vi "1 Optical Motion (with Velocity Plot).vi"() -> ()   [LabVIEW 2012]
doc: "This example shows how to use the Lucas Kanade Pyramid motion estimation VI to track features in a sequence of images in NI Vision. The VI reads the frames from an AVI file and tracks user specified features in the image from frame to frame."
uses:
  <vilib>/userdefined/High Color/IMAQdx.ctl
  <vilib>/vision/driver/NI_Vision_Acquisition_Software.lvlib
  <vilib>/vision/NI_Vision_Development_Module.lvlib
panel:
  out "Distance Array":dbl[](array[slide])=[0.2733994049757765, 0.23499957403887414, 0.19572823579546908, 0.3099445751011246, 0.800848062565794, 0.07985501092672606, 0.034294158969479405, 0.2777074897572326, 0.19929800724297095, 0.1271143119257122, 0.21415195112343915, 0.28639636417045206, 0.3114689873551136, 0.07118602059901899] caption="DistanceArray" scale=0.0..40.0
  in  "Select Points":bool caption="Click on the image and select the points to track. Press the <Ctrl> key while selecting  multiple points. Press the  \"Select Points\" button after  all points have been selected."
  in  "Options":T1={"Level"=4, "maxiteration"=20, "windowsize"=20, "threshold"=1.0}
  out "Image":T2(plugin-control)
  in  "Stop":bool
  # "My iphone is low resolution. You may need\nto experiment with these setting to make it\nwork correctly with your camera. Start by \ntweeking the Window Size"
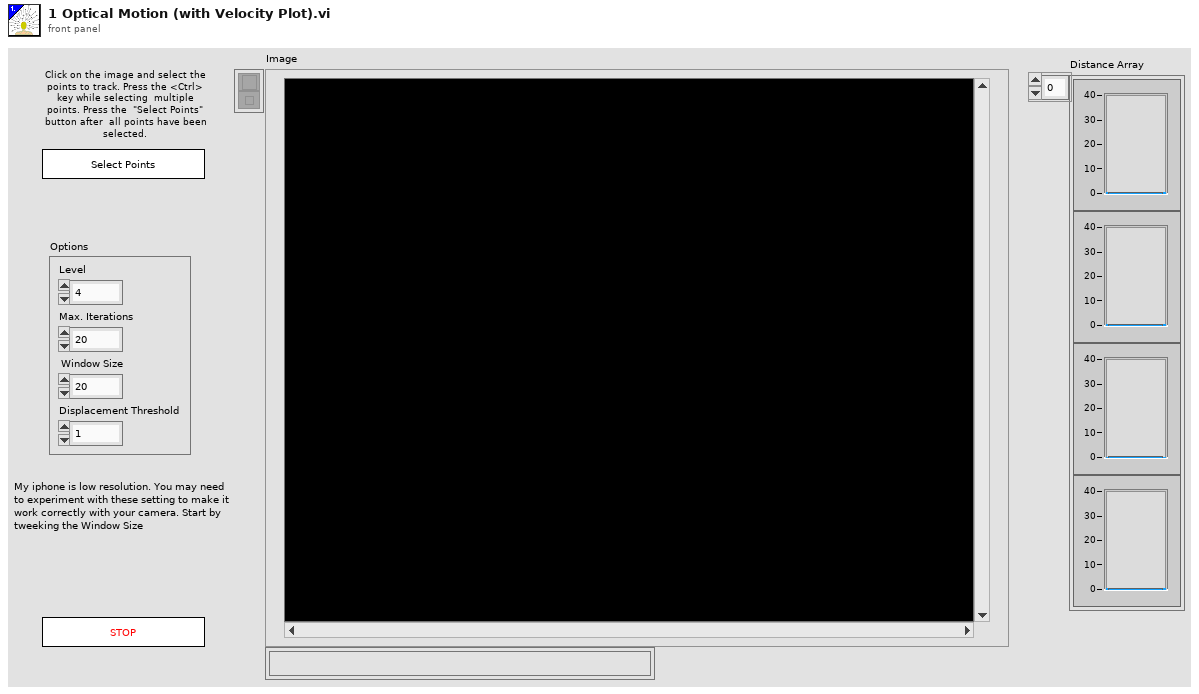
[diagram p1: front panel]
types:
  T1 = cluster{"Level":i32, "maxiteration":i32, "windowsize":i32, "threshold":dbl}
  T2 = typedef "IMAQ Image.ctl" = refnum<image>
  T3 = typedef "IMAQdx.ctl" = refnum<k21>
  T4 = cluster{"Global Rectangle":i32[], "Contours":cluster{"Contour Type":u32, "ROI Type":u32, "Points":i32[]}[]}
  T5 = typedef "ROI Descriptor" = cluster{"Global Rectangle":i32[], "Contours":cluster{"ID":enum32{"External", "Internal"}, "Type":u32, "Coordinates":i32[]}[]}
  T6 = typedef "IMAQ Point" = cluster{"X":sgl, "Y":sgl}
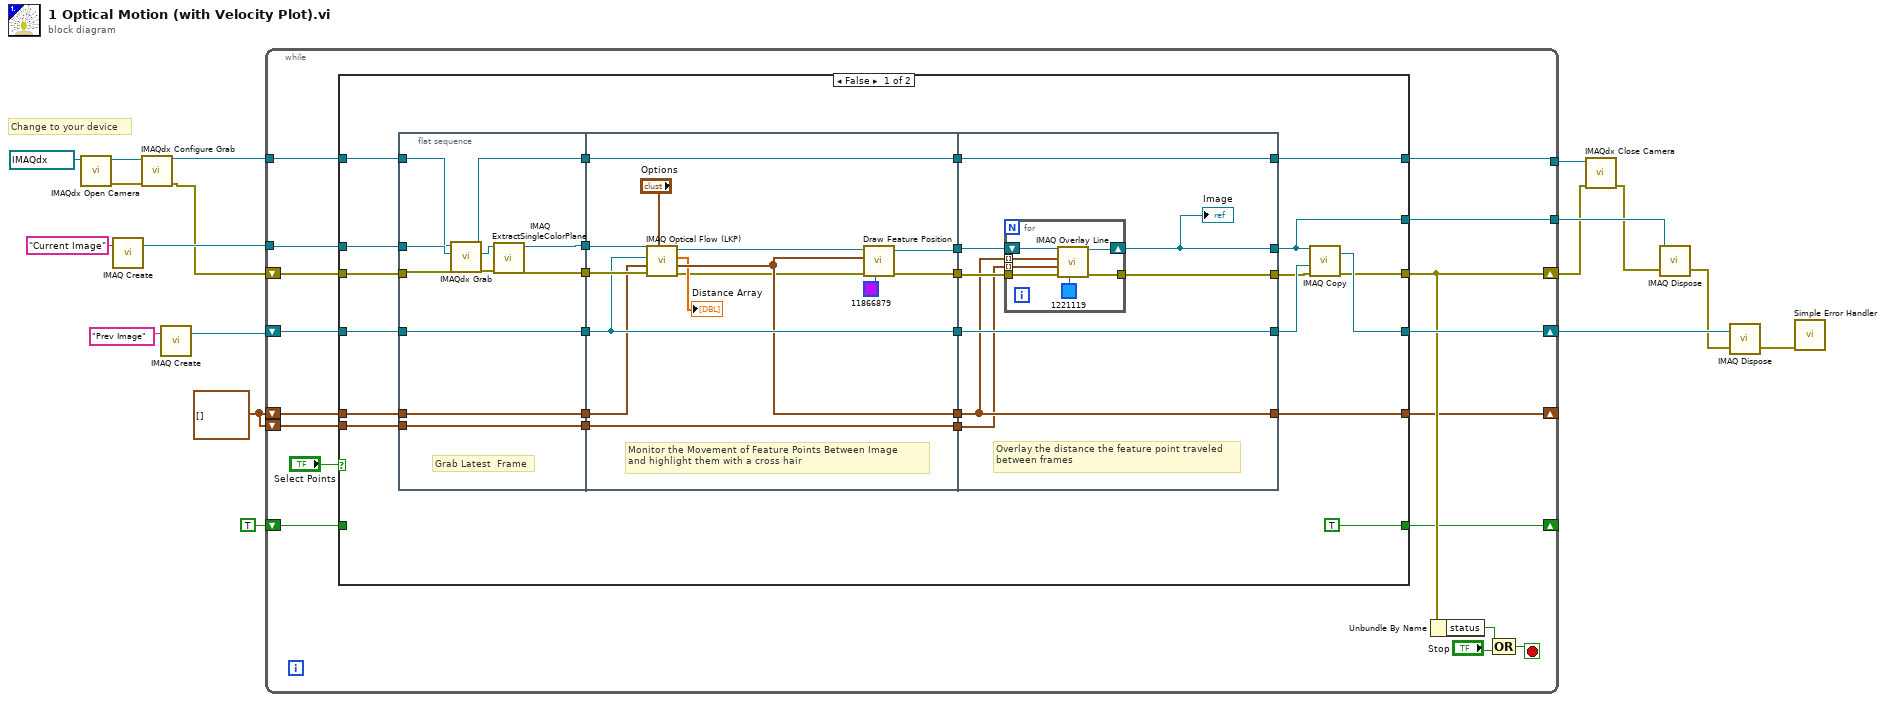
[diagram p0: block diagram]
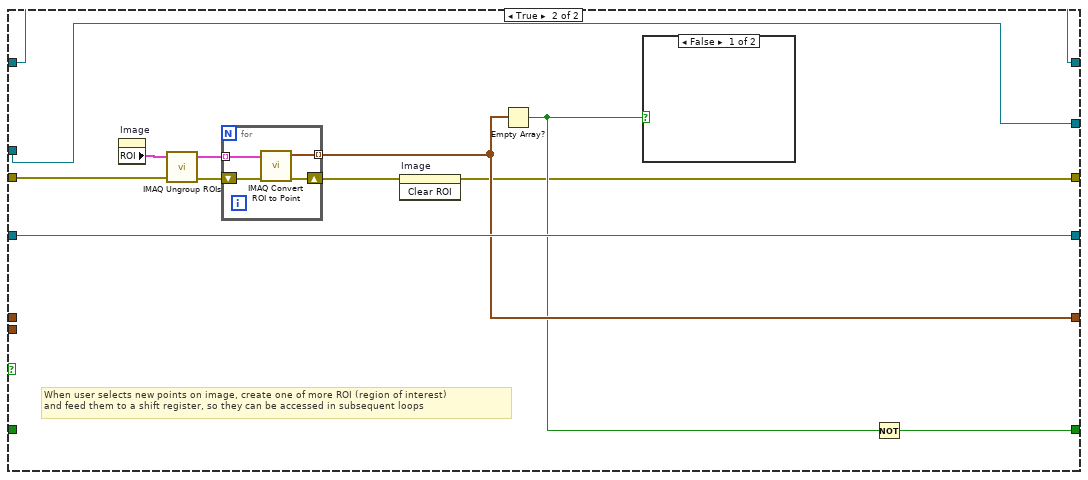
[diagram p2: hidden frame]
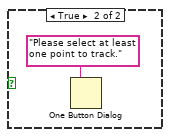
[diagram p3: hidden frame]
diagram:
  w8 = cluster{"X":sgl, "Y":sgl}[] [] ("Feature Points Out")
  # "Change to your device"
  n1 = call <vilib>:"IMAQdx Open Camera.vi"("Session In"=T3 "iPhone") -> ("error out"=w9:errorcluster, "Session Out"=w10:T3)  [unwired: 9 in]
  n2 = call "IMAQ Create"("Image Name"="Current Image") -> ("New Image"=w17:T2)  [unwired: 3 in, 2 out]
  n3 = call <vilib>:"IMAQdx Configure Grab.vi"("error in"=w9, "Session In"=w10) -> ("error out"=w2:errorcluster, "Session Out"=w1:T3)  [unwired: 8 in]
  n4 = call "IMAQ Create"("Image Name"="Prev Image") -> ("New Image"=w3:T2)  [unwired: 3 in, 2 out]
  n5 = while {
    tunnel: w17 -> [w23]
    shift-right: [w30] -> w14
    shift-left: w3 -> [w32]
    shift-right: [w27] -> _
    shift-left: w8 -> [w28]
    shift-right: [w25] -> _
    shift-left: TRUE -> [w24]
    shift-right: [w29] -> w7
    shift-left: w2 -> [w35]
    tunnel: [w22] -> w15
    tunnel: w1 -> [w21]
    tunnel: [w20] -> w12
    shift-left: w8 -> [w19]
    stop <- w33 stop-if-true
    n6 = case shown="False" "Select Points" {
      tunnel: w35 -> [w61 w108]
      tunnel: w23 -> [w60 w107]
      tunnel: w32 -> [w59 w113]
      tunnel: [w58 w113] -> w30
      tunnel: [w57 w104] -> w29
      tunnel: w28 -> [w56 _]
      tunnel: [w55 w106] -> w27
      tunnel: [TRUE w103] -> w25
      tunnel: w24 -> [_ _]
      tunnel: [w53 w107] -> w22
      tunnel: w21 -> [w52 w102]
      tunnel: [w51 w102] -> w20
      tunnel: w19 -> [w50 _]
      frame False {
        n7 = flat-sequence {
          tunnel: [w62] -> w48
          tunnel: w60 -> [w70]
          tunnel: w61 -> [w67]
          tunnel: w59 -> [w72]
          tunnel: [w72] -> w49
          tunnel: [w71] -> w46
          tunnel: w56 -> [w71]
          tunnel: [w65] -> w47
          tunnel: w52 -> [w69]
          tunnel: [w68] -> w45
          tunnel: [w64] -> w44
          tunnel: w50 -> [w64]
          tunnel: [w74] -> w43
          tunnel: [w85] -> w42
          tunnel: w49 -> [w85]
          tunnel: w48 -> [w86]
          tunnel: w47 -> [w83]
          tunnel: w46 -> [w80]
          tunnel: [w81] -> w41
          tunnel: [w82] -> w40
          tunnel: [w79] -> w39
          tunnel: w45 -> [w79]
          tunnel: w44 -> [w77]
          tunnel: [w77] -> w38
          tunnel: w43 -> [w91]
          tunnel: w42 -> [w94]
          tunnel: [w94] -> w37
          tunnel: w41 -> [w90]
          tunnel: [w90] -> w55
          tunnel: w40 -> [w92]
          tunnel: [w88] -> w53
          tunnel: [w93] -> w51
          tunnel: w39 -> [w93]
          tunnel: w38 -> [w89]
          tunnel: [w87] -> w36
          frame #0 {
            # "Grab Latest  Frame"
            n8 = call <vilib>:"IMAQdx Grab.vi"("error in"=w67, "Image In"=w70, "Session In"=w69) -> ("error out"=w63:errorcluster, "Image Out"=w66:T2, "Session Out"=w68:T3)  [unwired: 5 in, 1 out]
            n9 = call "IMAQ ExtractSingleColorPlane"("error in (no error)"=w63, "Image Src"=w66) -> ("error out"=w62:errorcluster, "Image Dst Out"=w65:T2)  [unwired: 8 in]
          }
          frame #1 {
            # "Monitor the Movement of Feature Points Between Image\nand highlight them with a cross hair"
            n10 = call "IMAQ Optical Flow (LKP)"("Options"="Options", "error in (no error)"=w86, "Feature Points In"=w80, "Previous Frame"=w85, "Current Frame"=w83) -> ("error out"=w73:errorcluster, "Feature Points Out"=w81:cluster{"X":sgl, "Y":sgl}[], "Distance Array"=→"Distance Array":dbl[], "Current Frame Out (dup)"=w76:T2)  [unwired: 1 in, 2 out]
            n11 = call "Draw Feature Position.vi"("Color"=u32 11866879, "Error In"=w73, "Feature Ponts"=w81, "Image"=w76) -> ("Error Out"=w74:errorcluster, "Image Out"=w82:T2)  [unwired: 6 out]
          }
          frame #2 {
            # "Overlay the distance the feature point traveled\nbetween frames"
            n12 = for {
              tunnel: w91 -> [w99]
              tunnel: [w98] -> w87
              tunnel: w90 -> [w96] mode=indexing
              tunnel: w89 -> [w95] mode=indexing
              shift-right: [w100] -> w88
              shift-left: w92 -> [w101]
              n13 = call "IMAQ Overlay Line"("Color"=u32 1221119, "error in (no error)"=w99, "End Point"=w95, "Start Point"=w96, "Image"=w101) -> ("error out"=w98:errorcluster, "Image Out"=w100:T2)  [unwired: 5 in]
            }
            "Image" <- w88
          }
        }
        n14 = call "IMAQ Copy"("error in (no error)"=w36, "Image Dst"=w37, "Image Src"=w53) -> ("error out"=w57:errorcluster, "Image Dst Out"=w58:T2)  [unwired: 3 out]
      }
      frame True {
        # "When user selects new points on image, create one of more ROI (region of interest)\nand feed them to a shift register, so they can be accessed in subsequent loops"
        n15 = property on="Image" class="ImageControl"() -> ("ROI"=w112:T4)  [unwired: 2 in, 2 out]
        n16 = call "IMAQ Ungroup ROIs"("error in (no error)"=w108, "ROI Descriptor"=w112) -> ("error out"=w111:errorcluster, "ROI Descriptors out"=w110:T5[])  [unwired: 2 out]
        n17 = for {
          shift-right: [w115] -> w109
          shift-left: w111 -> [w118]
          tunnel: w110 -> [w117] mode=indexing
          tunnel: [w116] -> w106 mode=indexing
          n18 = call "IMAQ Convert ROI to Point"("error in (no error)"=w118, "ROI Descriptor"=w117) -> ("error out"=w115:errorcluster, "Point"=w116:T6)  [unwired: 7 out]
        }
        n19 = invoke on="Image" class="ImageControl" method="Clear ROI"(error in=w109) -> (error out=w104:errorcluster)  [unwired: 2 in, 2 out]
        n20 = Empty Array?(array=w106) -> (empty?=w105:bool)
        n21 = case shown="False" w105 {
          frame False {
          }
          frame True {
            n22 = One Button Dialog(message="Please select at least one point to track.") -> ()  [unwired: 2 out]
          }
        }
        n23 = Not(x=w105) -> (.not. x?=w103:bool)
      }
    }
    n24 = Unbundle By Name(w29) -> ("status"=w31:bool)
    n25 = Compound Arithmetic op=OR(w31, "Stop") -> (w33:bool)
  }
  n26 = call <vilib>:"IMAQdx Close Camera.vi"("error in"=w7, "Session In"=w12) -> ("error out"=w6:errorcluster)  [unwired: 9 in]
  n27 = call "IMAQ Dispose"("Image"=w15, "error in (no error)"=w6) -> ("error out"=w5:errorcluster)  [unwired: 1 in, 3 out]
  n28 = call "IMAQ Dispose"("Image"=w14, "error in (no error)"=w5) -> ("error out"=w4:errorcluster)  [unwired: 1 in, 3 out]
  n29 = call <vilib>:"Simple Error Handler.vi"("error in (no error)"=w4) -> ()  [unwired: 1 in, 8 out]
